vi "S2C_Shared_Proc_ManageLog.vi"(5 "Local?":bool, 7 "Command":string, 8 "Error In":errorcluster, 10 "Refs":string[][](array[string]), 11 "Data In":string) -> (0 "Error Out":errorcluster, 3 "Data Out":string)   [LabVIEW 2015]
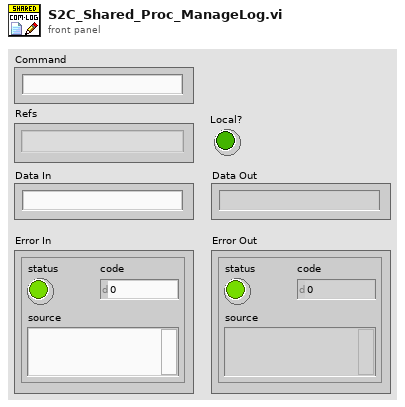
[diagram p1: front panel]
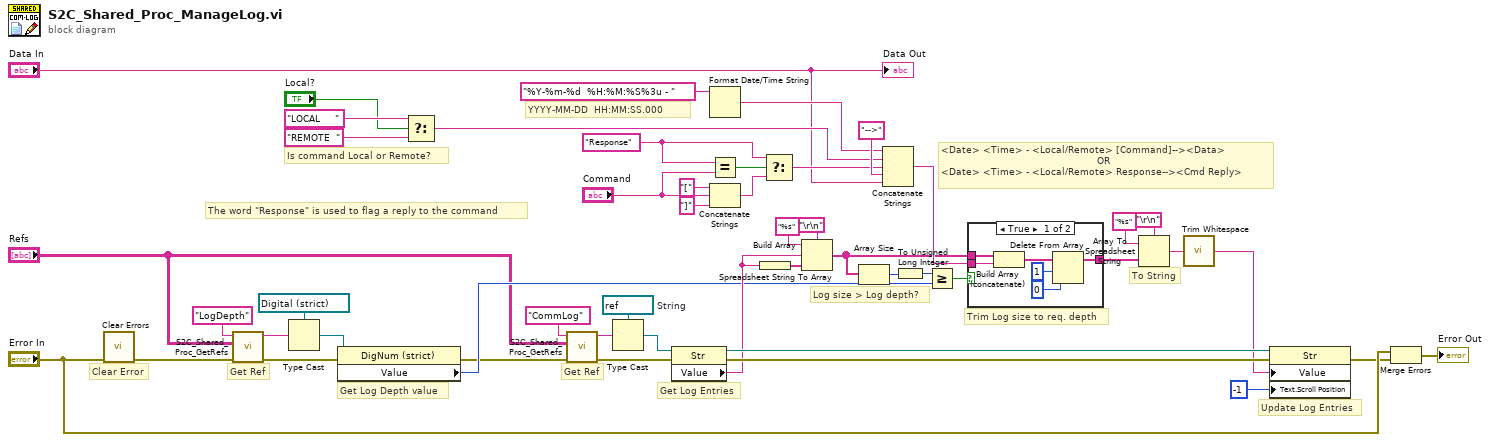
[diagram p0: block diagram]
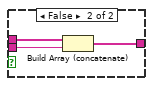
[diagram p2: hidden frame]
diagram:
  w13 = refnum<vi> refnum  # String
  w23 = "Response" ("y")
  # "YYYY-MM-DD  HH:MM:SS.000"
  # "The word \"Response\" is used to flag a reply to the command"
  # "Update Log Entries"
  # "<Date> <Time> - <Local/Remote> [Command]--><Data>\n                                                    OR\n<Date> <Time> - <Local/Remote> Response--><Cmd Reply>"
  # "To String"
  # "Trim Log size to req. depth"
  # "Log size > Log depth?"
  # "Get Log Entries"
  # "Get Ref"
  # "Is command Local or Remote?"
  # "Get Log Depth value"
  # "Get Ref"
  # "Clear Error"
  n1 = call <vilib>:"Clear Errors.vi"("error in (no error)"="Error In") -> ("error out"=w5:errorcluster)  [unwired: 5 in, 1 out]
  n2 = call "S2C_Shared_Proc_GetRefs.vi"("Error In"=w5, "Refs"="Refs", "Label"="LogDepth") -> ("Error Out"=w4:errorcluster, "Reference"=w6:string)  [unwired: 7 in]
  n3 = Type Cast(type=refnum<vi> refnum ("LogDepth"), x=w6) -> (*(type *) &x=w3:refnum<vi>)
  n4 = property class="DigNum (strict)"(reference=w3, error in=w4) -> (error out=w10:errorcluster, "Value"=w36:u32)  [unwired: 1 out]
  n5 = Select(t="LOCAL     " ("y"), s="Local?", f="REMOTE  " ("y")) -> (s? t:f=w17:string)
  n6 = call "S2C_Shared_Proc_GetRefs.vi"("Error In"=w10, "Refs"="Refs", "Label"="CommLog") -> ("Error Out"=w8:errorcluster, "Reference"=w12:string)  [unwired: 7 in]
  n7 = Type Cast(type=w13, x=w12) -> (*(type *) &x=w9:refnum<vi>)
  n8 = property class="Str"(reference=w9, error in=w8) -> (reference out=w46:refnum<vi>, error out=w45:errorcluster, "Value"=w44:string)
  n9 = Format Date/Time String(time format string (%c)="%Y-%m-%d  %H:%M:%S%3u - ") -> (date/time string=w18:string)  [unwired: 2 in]
  n10 = Equal?(x=w23, y="Command") -> (x = y?=w25:bool)
  n11 = Concatenate Strings("[" ("string"), "Command", "]" ("string")) -> (w22:string)
  n12 = Build Array(w44) -> (w43:string[])
  n13 = Select(t=w23, s=w25, f=w22) -> (s? t:f=w24:string)
  n14 = Spreadsheet String To Array(delimiter (Tab)="\r\n", format string="%s", spreadsheet string=w44, array type (2D Dbl)=w43) -> (array=w37:string[])
  n15 = Array Size(array=w37) -> (size(s)=w39:i32)
  n16 = Concatenate Strings(w18, w17, w24, "-->" ("string"), "Data In") -> (w40:string)
  n17 = To Unsigned Long Integer(number=w39) -> (unsigned 32bit integer=w35:u32)
  n18 = Greater Or Equal?(x=w35, y=w36) -> (x >= y?=w38:bool)
  n19 = case shown="True" w38 {
    tunnel: w40 -> [w54 w57]
    tunnel: w37 -> [w55 w58]
    tunnel: [w50 w56] -> w34
    frame True {
      n20 = Build Array (concatenate)(w55, w54) -> (w53:string[])
      n21 = Delete From Array(array=w53, length=1, index=0) -> (array with subset deleted=w50:string[])  [unwired: 1 out]
    }
    frame False {
      n22 = Build Array (concatenate)(w58, w57) -> (w56:string[])
    }
  }
  n23 = Array To Spreadsheet String(delimiter (Tab)="\r\n", array=w34, 3:"%s" ("format string")) -> (spreadsheet string=w31:string)
  n24 = call <vilib>:"Trim Whitespace.vi"("string"=w31) -> ("trimmed string"=w28:string)  [unwired: 1 in]
  n25 = property class="Str"(reference=w46, error in=w45, "Value"=w28, "Text.Scroll Position"=-1) -> (error out=w30:errorcluster)  [unwired: 1 out]
  n26 = Merge Errors("Error In", w30) -> (→"Error Out":errorcluster)
  "Data Out" <- "Data In"
